vi "AppState.vi"() -> ()   [LabVIEW 2013]
panel:
  in  "AppState":u16
  # "Idle: 0\nCalibration: 1\nMesure: 2"
  # "Vidange: 3"
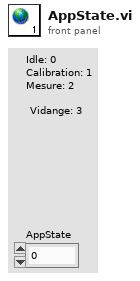
[diagram p1: front panel]
diagram:
